vi "Wavelet Packet - Entropy Selection.vi"() -> ()   [LabVIEW 2023]
doc: "This example shows different methods that you can use for entropy computation. The best wavelet packet tree is plotted in this example. This example shows that different methods may generate different best trees.\n\n<b>Instructions:</b>\n1) Run this VI.\n2) Observe the best trees for the signal with different entropy settings."
uses:
  <vilib>/addons/Wavelet Analysis/wavelet packet.llb/WA WP Decomposition (Waveform).vi
  <vilib>/addons/_Advanced Signal Processing/NI_AdvSigProcWA.lvlib
panel:
  in  "Data":u16(ring)=115 items=["1D Example Data"=100, "-"=101, "Doppler"=102, "HOP"=103, "TF Sine"=104, "Noisy Doppler"=105, "Sea Temperature"=106, "Sp500"=107, "Power Line"=108, "Engine Knocking"=109, "HeaviSine"=110, "Bumps"=111, "Blocks"=112, "Piece Regular"=113, "HypChirps"=114, "LinChirps"=115, "Chirps"=116, "Piece Polynomial"=117, "ECG"=131, "-"=118, "2D Example Data"=119, "-"=120, "Finger Print (Image)"=121, "Iris Flower (Image)"=122, "Mammogram (Image)"=123, "Lake (Image)"=127, "Two Can 1 (Image)"=132, "Two Can 2 (Image)"=133, "Camera Man (Image)"=134]
  in  "Levels":i32=4
  in  "stop":bool
  out "Signal":waveform(dbl)(graph)
  out "Best Tree":picture
  in  "Entropy":T1={"Entropy Type"=0, "Optional Parameter"=1.0} {"Entropy Type" items=["shannon", "threshold", "sure", "norm", "energy"]}
  in  "Wavelet":u16(ring)=3 items=["db02"=0, "db03"=1, "db04"=2, "db05"=3, "db06"=4, "db07"=5, "db08"=6, "db09"=7, "db10"=8, "db11"=9, "db12"=10, "db13"=11, "db14"=12, "Haar"=13, "bior1_3"=14, "bior1_5"=15, "bior2_2"=16, "bior2_4"=17, "bior2_6"=18, "bior2_8"=19, "bior3_1"=20, "bior3_3"=21, "bior3_5"=22, "bior3_7"=23, "bior3_9"=24, "bior4_4 (FBI)"=25, "bior5_5"=38, "bior6_8"=39, "coif1"=26, "coif2"=27, "coif3"=28, "coif4"=29, "coif5"=30, "sym2"=31, "sym3"=32, "sym4"=33, "sym5"=34, "sym6"=35, "sym7"=36, "sym8"=37]
  # "Overview: Shows different methods that you can use for entropy computation. The best wavelet packet tree is plotted in this example. \nRequirements: LabVIEW Full Development System, Advanced Signal Processing Toolkit\nInstructions: \n1. Run this VI.\n2. Observe the best trees for the signal with different entropy settings.\n3. Click Stop to stop the VI."
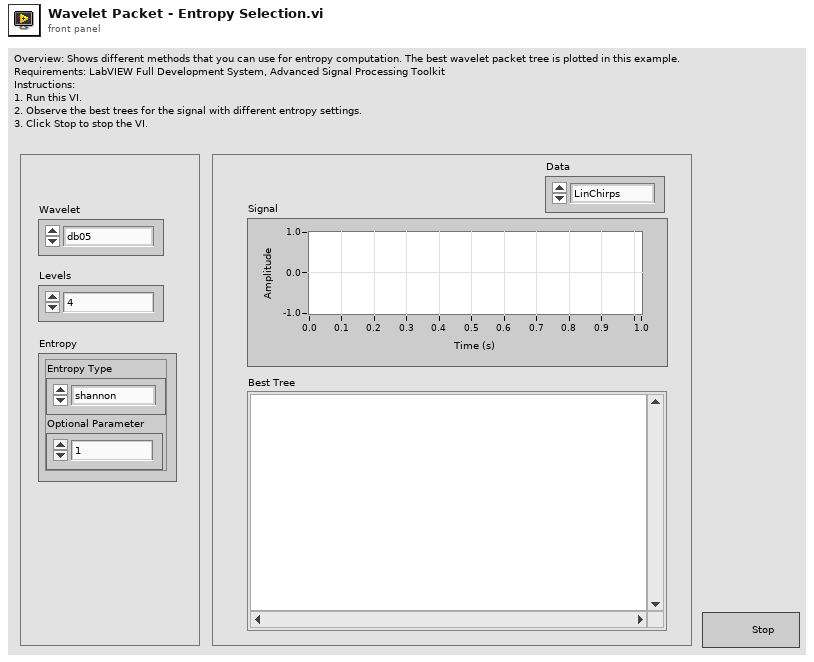
[diagram p1: front panel]
types:
  T1 = cluster{"Entropy Type":u16, "Optional Parameter":dbl}
  T2 = typedef "NI_AdvSigProcWA.lvlib/WA Generic Ref.ctl" = cluster{"ref":u64, "t0":timestamp, "dt":dbl}
  T3 = typedef "LVBoundsTypeDef.ctl" = cluster{"Width":u32, "Height":u32}
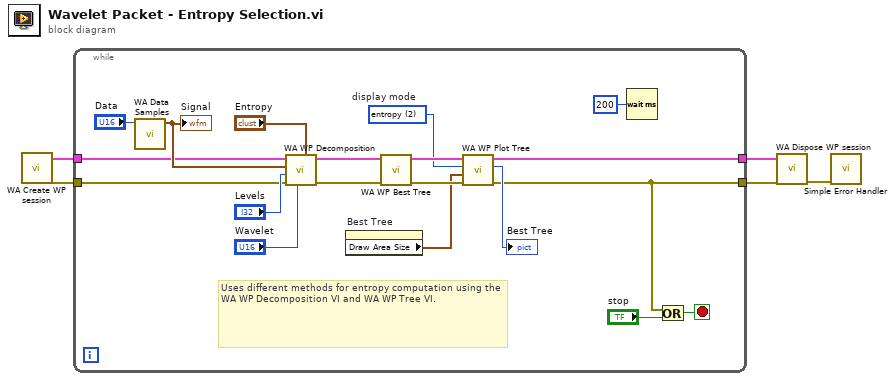
[diagram p0: block diagram]
diagram:
  n1 = call <vilib>:"WA Create WP session.vi"() -> ("error out"=w4:errorcluster, "WP session out"=w5:T2)  [unwired: 1 in, 9 out]
  n2 = while {
    tunnel: w5 -> [w10]
    tunnel: w4 -> [w9]
    tunnel: [w8] -> w3
    tunnel: [w6] -> w2
    stop <- w12 stop-if-true
    w15 = u16 2 items=["node path", "(depth, pos)", "entropy"]  # display mode
    # "Uses different methods for entropy computation using the WA WP Decomposition VI and WA WP Tree VI."
    n3 = call <vilib>:"WA Data Samples.vi"("data"="Data") -> ("signal"=w14:waveform(dbl))  [unwired: 10 out]
    "Signal" <- w14
    n4 = call-poly <vilib>:"WA WP Decomposition.vi"("entropy"="Entropy", "wavelet"="Wavelet", "error in (no error)"=w9, "levels"="Levels", "signal"=w14, "WP session"=w10) -> ("error out"=w23:errorcluster, "WP session out"=w24:T2)  [unwired: 4 out]
    n5 = property on="Best Tree" class="Pict"() -> ("Draw Area Size"=w16:T3)  [unwired: 2 in, 2 out]
    n6 = call <vilib>:"WA WP Best Tree.vi"("error in (no error)"=w23, "WP session"=w24) -> ("error out"=w21:errorcluster, "WP session out"=w22:T2)  [unwired: 8 out]
    n7 = call <vilib>:"WA WP Plot Tree.vi"("error in (no error)"=w21, "draw area size"=w16, "display mode"=w15, "WP session"=w22) -> ("error out"=w6:errorcluster, "tree plot"=→"Best Tree":picture, "WP session out"=w8:T2)  [unwired: 5 out]
    n8 = Wait (ms)(milliseconds to wait=u32 200 ("millisecond multiple")) -> ()  [unwired: 1 out]
    n9 = Or(x=w6, y="stop") -> (x .or. y?=w12:bool)
  }
  n10 = call <vilib>:"WA Dispose WP session.vi"("error in (no error)"=w2, "WP session"=w3) -> ("error out"=w1:errorcluster)  [unwired: 9 out]
  n11 = call <vilib>:"Simple Error Handler.vi"("error in (no error)"=w1) -> ()  [unwired: 1 in, 8 out]
